vi "Add UEGO card.vi"(8 "error in (no error)":errorcluster, 10 "FPGA Item Name":string, 11 "Node Ptr":u64 format="%.0x") -> (0 "error out":errorcluster)   [LabVIEW 2014, in "SLSC configuration System Explorer.lvlib"]
uses:
  SLSC configuration System Explorer.lvlib
  Shared/Constants.vi
  Shared/SLSC configuration Shared.lvlib
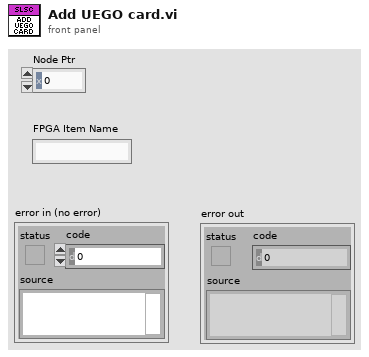
[diagram p1: front panel]
types:
  T1 = typedef "SLSC configuration Shared.lvlib/Card Position.ctl" = cluster{"Rack #":u8, "Slot #":T2}
  T2 = typedef "SLSC configuration Shared.lvlib/Slot #.ctl" = u8
  T3 = typedef "Custom Device API.lvlib/Custom Device Item Ref.ctl" = u64
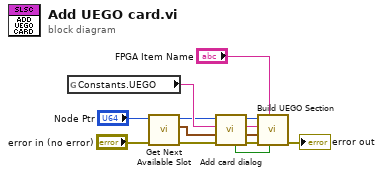
[diagram p0: block diagram]
diagram:
  n1 = global read "Constants.vi" "Constants.UEGO"() -> (w9:string)
  n2 = call "Get Next Available Slot.vi"("error in (no error)"="error in (no error)", "Device Ref in"="Node Ptr") -> ("error out"=w5:errorcluster, "Next Open Slot"=w4:T1, "Device Ref out"=w2:T3)  [unwired: 7 in]
  n3 = call "Add card dialog.vi"("error in (no error)"=w5, "Card Position"=w4, "Card Type in"=w9, "Node Ptr"=w2) -> ("error out"=w13:errorcluster, "Card Position out"=w10:T1, "Name out"=w12:string, "Node Ptr out"=w11:u64, "Cancelled?"=w7:bool)  [unwired: 3 in]
  n4 = call "Build UEGO Section.vi"("Cancelled?"=w7, "FPGA Item Name"="FPGA Item Name", "error in (no error)"=w13, "Card Position in"=w10, "Name in"=w12, "Node Ptr in"=w11) -> ("error out"=→"error out":errorcluster)  [unwired: 5 in]
